vi "Calculate F(x) - outputs.vi"() -> ()   [LabVIEW 2023]
panel:
  out "f(x)":dbl=-16.933324334395763
  out "val1":dbl
  out "Waveform Graph 2":dbl[](graph)
  out "Waveform Graph":dbl[](graph)
  out "Output Array":dbl[][](array[numeric])
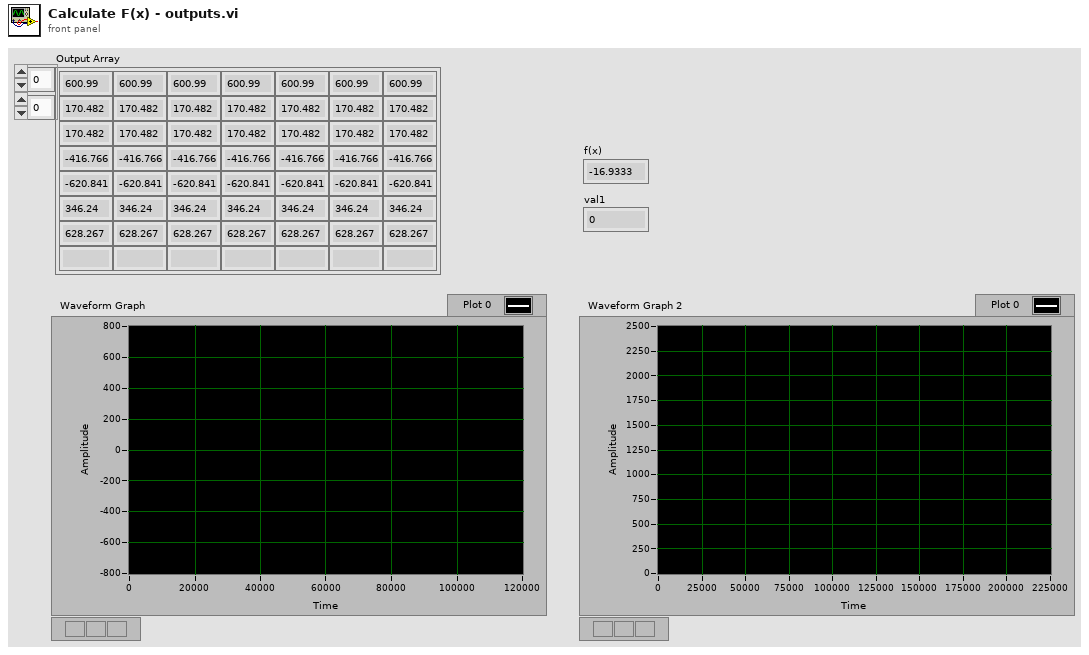
[diagram p1: front panel]
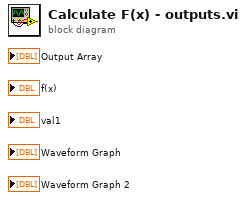
[diagram p0: block diagram]
diagram:
